vi "DMA.Write Single.vi"(8 "error in (no error)":errorcluster, 9 "timeout ms (1000)":u32=1000, 10 "DMA Transfer Spec":T1 {"Block Descriptors"."next descriptor ptr" format="%08x"; "Block Descriptors"."data size" format="%08x"; "Block Descriptors"."data ptr (upper)" format="%08x"; "Block Descriptors"."data ptr (lower)" format="%08x"; "Block Descriptors"."descriptor ptr (aligned)" format="%08x"; "Block Descriptors"."descriptor size" format="%08x"; "Block Descriptors"."descriptor ptr (VISA)" format="%08x"; "RFM Address" format="%08x"}, 11 "GE 5565PIORC":refnum<class "GE 5565PIORC Old.lvclass">) -> (0 "error out":errorcluster, 1 "Timed out?":bool, 2 "DMA Transfer Spec out":T1 {"Block Descriptors"."next descriptor ptr" format="%08x"; "Block Descriptors"."data size" format="%08x"; "Block Descriptors"."data ptr (upper)" format="%08x"; "Block Descriptors"."data ptr (lower)" format="%08x"; "Block Descriptors"."descriptor ptr (aligned)" format="%08x"; "Block Descriptors"."descriptor size" format="%08x"; "Block Descriptors"."descriptor ptr (VISA)" format="%08x"; "RFM Address" format="%08x"}, 3 "GE 5565PIORC out":refnum<class "GE 5565PIORC Old.lvclass">)   [LabVIEW 2016, in "GE 5565PIORC Old.lvclass"]
uses:
  GE 5565PIORC Old.lvclass
  Controls/DMA Transfer Spec.ctl
  Controls/DMA Block Descriptor.ctl
  GE 5565PIORC Old.lvclass/GE 5565PIORC Old.ctl
  Registers/Local Configuration.DMACSR0.DMA Start.Set.vi
  Interrupts/Wait for PXI Interrupt Events.vi
  Registers/Local Configuration.DMACSR0.DMA Clear Interrupt.Set.vi
  <vilib>/Utility/error.llb/Clear Errors.vi
  DMA.Transfer Size.vi
  Registers/Local Configuration.PCI Address.Set.vi
  Registers/Local Configuration.DMADPR0.First Descriptor Address.Set.vi
  DMA.Scatter-Gather.Link Block Descriptors.vi
  DMA.Scatter-Gather.Commit Blocks.vi
  Registers/Local Configuration.Local Address.Set.vi
  Registers/Local Configuration.Transfer Size.Set.vi
  Registers/Local Configuration.DMADPR0.Transfer Direction.Set.vi
  Registers/Local Configuration.DMAMODE0.Scatter-Gather Enable.Set.vi
  Binary Operations/Set Bits.vi
  Binary Operations/Set Bits U32.vi
  Registers/Local Configuration.Get Register Offset.vi
  Binary Operations/Get Bits.vi
  Binary Operations/Get Bits U32.vi
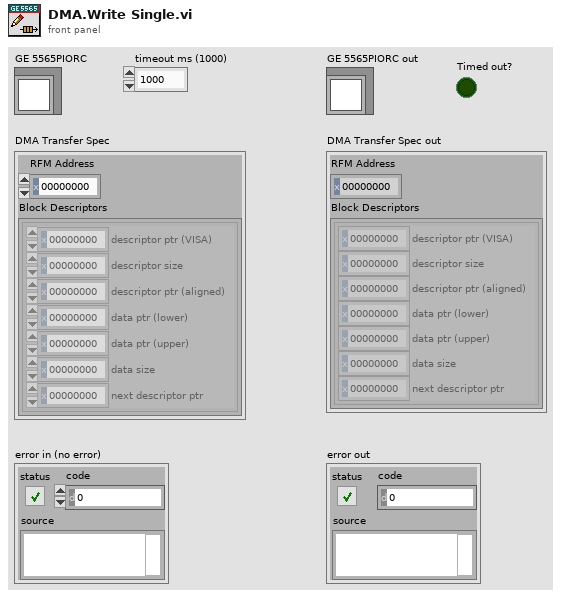
[diagram p1: front panel]
types:
  T1 = typedef "GE 5565PIORC Old.lvclass/DMA Transfer Spec.ctl" = cluster{"RFM Address":u32, "Block Descriptors":T2[]}
  T2 = typedef "GE 5565PIORC Old.lvclass/DMA Block Descriptor.ctl" = cluster{"descriptor ptr (VISA)":u32, "descriptor size":u32, "descriptor ptr (aligned)":u32, "data ptr (lower)":u32, "data ptr (upper)":u32, "data size":u32, "next descriptor ptr":u32}
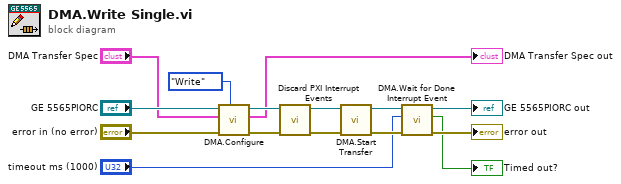
[diagram p0: block diagram]
diagram:
  n1 = call "DMA.Configure.vi"("Transfer Direction"=enum16{"Write", "Read"}."Write", "error in (no error)"="error in (no error)", "DMA Transfer Spec"="DMA Transfer Spec", "GE 5565PIORC"="GE 5565PIORC") -> ("error out"=w5:errorcluster, "DMA Transfer Spec out"=→"DMA Transfer Spec out":T1, "GE 5565PIORC out"=w4:refnum<class "GE 5565PIORC Old.lvclass">)  [unwired: 5 in]
  n2 = call "Discard PXI Interrupt Events.vi"("error in (no error)"=w5, "GE 5565PIORC in"=w4) -> ("error out"=w6:errorcluster, "GE 5565PIORC out"=w7:refnum<class "GE 5565PIORC Old.lvclass">)  [unwired: 8 in]
  n3 = call "DMA.Start Transfer.vi"("error in (no error)"=w6, "GE 5565PIORC"=w7) -> ("error out"=w11:errorcluster, "GE 5565PIORC out"=w12:refnum<class "GE 5565PIORC Old.lvclass">)  [unwired: 8 in]
  n4 = call "DMA.Wait for Done Interrupt Event.vi"("error in (no error)"=w11, "timeout ms (1000)"="timeout ms (1000)", "GE 5565PIORC"=w12) -> ("error out"=→"error out":errorcluster, "Timed out?"=→"Timed out?":bool, "GE 5565PIORC out"=→"GE 5565PIORC out":refnum<class "GE 5565PIORC Old.lvclass">)  [unwired: 6 in]
